vi "Format String to Numeric.vi"(4 "Response":string, 5 "Ignore String":string, 6 "Type":T2, 7 "Data Parameters.List":string[](array[string]), 8 "error in (no error)":errorcluster, 9 "Channel Type":T1, 10 "Format String":string, 11 "Expected String":string) -> (0 "error out":errorcluster, 2 "Value":dbl, 3 "remaining string":string)   [LabVIEW 2013, in "Instrument Addon Engine.lvlib"]
uses:
  Instrument Addon Engine.lvlib
  Shared/Types/Type Cast Type.ctl
  Shared/Types/Data Channel Type.ctl
  Shared/Instrument Addon Shared.lvlib
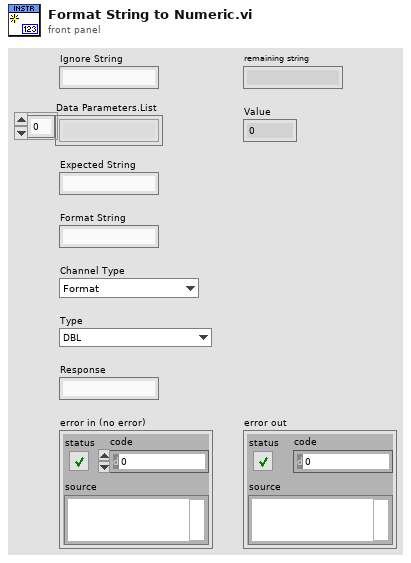
[diagram p1: front panel]
types:
  T1 = typedef "Instrument Addon Shared.lvlib/Data Channel Type.ctl" = enum16{"Format", "Comparison", "Type Cast", "Enumerated List"}
  T2 = typedef "Instrument Addon Shared.lvlib/Type Cast Type.ctl" = enum16{"DBL", "SGL", "U64", "U32", "U16", "U8", "I64", "I32", "I16", "I8"}
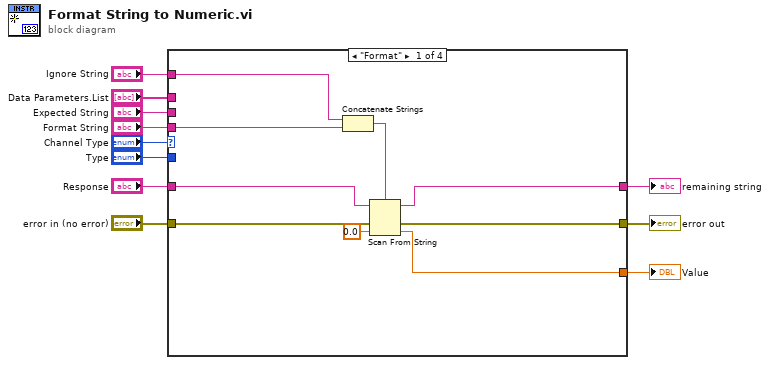
[diagram p0: block diagram]
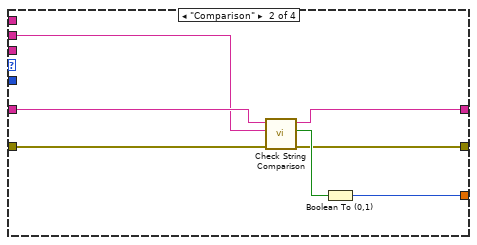
[diagram p2: hidden frame]
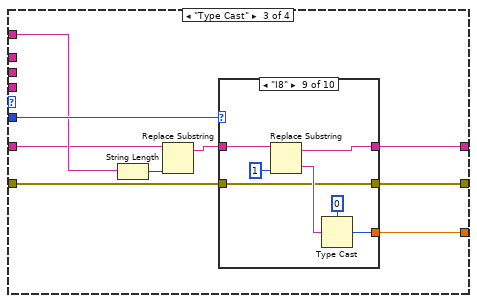
[diagram p3: hidden frame]
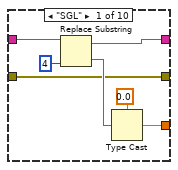
[diagram p4: hidden frame]
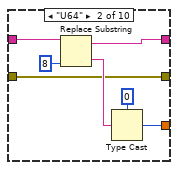
[diagram p5: hidden frame]
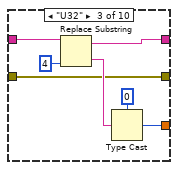
[diagram p6: hidden frame]
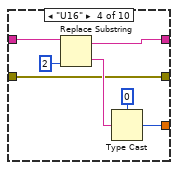
[diagram p7: hidden frame]
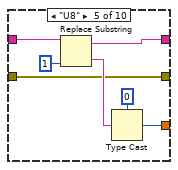
[diagram p8: hidden frame]
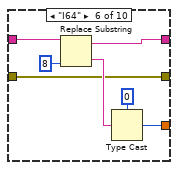
[diagram p9: hidden frame]
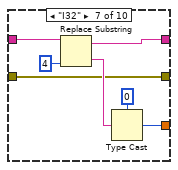
[diagram p10: hidden frame]
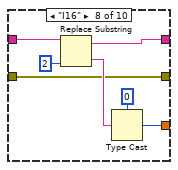
[diagram p11: hidden frame]
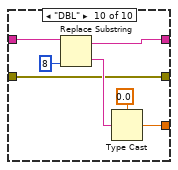
[diagram p12: hidden frame]
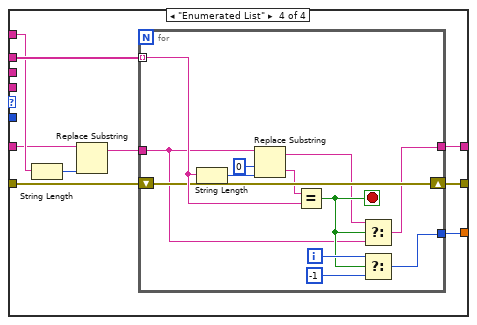
[diagram p13: hidden frame]
diagram:
  n1 = case shown="\"Format\"" "Channel Type" {
    tunnel: [w19 w27 w35 w113] -> w9
    tunnel: "Response" -> [w20 w26 w31 w108]
    tunnel: [w18 w24 w36 w111] -> w3
    tunnel: "Ignore String" -> [w16 _ w32 w109]
    tunnel: "Format String" -> [w15 _ _ _]
    tunnel: "error in (no error)" -> [w14 w22 w29 w115]
    tunnel: [w13 w21 w33 w112] -> w6
    tunnel: "Expected String" -> [_ w25 _ _]
    tunnel: "Type" -> [_ _ w34 _]
    tunnel: "Data Parameters.List" -> [_ _ _ w114]
    frame "Format" {
      n2 = Concatenate Strings(w16, w15) -> (w12:string)
      n3 = Scan From String(format string=w12, input string=w20, error in=w14, default 1=0.0 ("default value 1")) -> (remaining string=w18:string, error out=w13:errorcluster, output 1=w19:dbl)  [unwired: 1 in, 1 out]
    }
    frame "Comparison" {
      n4 = call "Check String Comparison.vi"("error in (no error)"=w22, "Expected String"=w25, "String"=w26) -> ("error out"=w21:errorcluster, "Found?"=w23:bool, "string out"=w24:string)  [unwired: 6 in]
      n5 = Boolean To (0,1)(Boolean=w23) -> (0, 1=w27:i16)
    }
    frame "Type Cast" {
      n6 = String Length(string=w32) -> (length=w28:i32)
      n7 = Replace Substring(2:w28, 5:w31) -> (1:w30:string)  [unwired: 2 in, 1 out]
      n8 = case shown="\"I8\"" w34 {
        tunnel: w30 -> [w43 w50 w57 w64 w71 w78 w85 w92 w99 w106]
        tunnel: [w42 w49 w56 w63 w70 w77 w84 w91 w98 w105] -> w36
        tunnel: [w38 w45 w52 w59 w66 w73 w80 w87 w94 w101] -> w35
        tunnel: [w37 w44 w51 w58 w65 w72 w79 w86 w93 w100] -> w33
        tunnel: w29 -> [w37 w44 w51 w58 w65 w72 w79 w86 w93 w100]
        frame "SGL" {
          n9 = Replace Substring(2:4 ("length (len. of substring)"), 5:w43) -> (0:w40:string, 1:w42:string)  [unwired: 2 in]
          n10 = Type Cast(type=sgl 0.0, x=w40) -> (*(type *) &x=w38:sgl)
        }
        frame "U64" {
          n11 = Replace Substring(2:8 ("length (len. of substring)"), 5:w50) -> (0:w47:string, 1:w49:string)  [unwired: 2 in]
          n12 = Type Cast(type=u64 0, x=w47) -> (*(type *) &x=w45:u64)
        }
        frame "U32" {
          n13 = Replace Substring(2:4 ("length (len. of substring)"), 5:w57) -> (0:w54:string, 1:w56:string)  [unwired: 2 in]
          n14 = Type Cast(type=u32 0, x=w54) -> (*(type *) &x=w52:u32)
        }
        frame "U16" {
          n15 = Replace Substring(2:2 ("length (len. of substring)"), 5:w64) -> (0:w61:string, 1:w63:string)  [unwired: 2 in]
          n16 = Type Cast(type=u16 0, x=w61) -> (*(type *) &x=w59:u16)
        }
        frame "U8" {
          n17 = Replace Substring(2:1 ("length (len. of substring)"), 5:w71) -> (0:w68:string, 1:w70:string)  [unwired: 2 in]
          n18 = Type Cast(type=u8 0, x=w68) -> (*(type *) &x=w66:u8)
        }
        frame "I64" {
          n19 = Replace Substring(2:8 ("length (len. of substring)"), 5:w78) -> (0:w75:string, 1:w77:string)  [unwired: 2 in]
          n20 = Type Cast(type=i64 0, x=w75) -> (*(type *) &x=w73:i64)
        }
        frame "I32" {
          n21 = Replace Substring(2:4 ("length (len. of substring)"), 5:w85) -> (0:w82:string, 1:w84:string)  [unwired: 2 in]
          n22 = Type Cast(type=0, x=w82) -> (*(type *) &x=w80:i32)
        }
        frame "I16" {
          n23 = Replace Substring(2:2 ("length (len. of substring)"), 5:w92) -> (0:w89:string, 1:w91:string)  [unwired: 2 in]
          n24 = Type Cast(type=i16 0, x=w89) -> (*(type *) &x=w87:i16)
        }
        frame "I8" {
          n25 = Replace Substring(2:1 ("length (len. of substring)"), 5:w99) -> (0:w96:string, 1:w98:string)  [unwired: 2 in]
          n26 = Type Cast(type=i8 0, x=w96) -> (*(type *) &x=w94:i8)
        }
        frame "DBL" {
          n27 = Replace Substring(2:8 ("length (len. of substring)"), 5:w106) -> (0:w103:string, 1:w105:string)  [unwired: 2 in]
          n28 = Type Cast(type=0.0, x=w103) -> (*(type *) &x=w101:dbl)
        }
      }
    }
    frame "Enumerated List" {
      n29 = String Length(string=w109) -> (length=w110:i32)
      n30 = Replace Substring(2:w110, 5:w108) -> (1:w107:string)  [unwired: 2 in, 1 out]
      n31 = for {
        shift-right: [w123] -> w112
        shift-left: w115 -> [w123]
        tunnel: w114 -> [w127] mode=indexing
        tunnel: w107 -> [w118]
        tunnel: [w124] -> w113
        tunnel: [w116] -> w111
        i -> [w126]
        stop <- w119 stop-if-true
        n32 = String Length(string=w127) -> (length=w122:i32)
        n33 = Replace Substring(2:w122, 3:0 ("offset (0)"), 5:w118) -> (0:w120:string, 1:w117:string)  [unwired: 1 in]
        n34 = Equal?(x=w120, y=w127) -> (x = y?=w119:bool)
        n35 = Select(t=w117, s=w119, f=w118) -> (s? t:f=w116:string)
        n36 = Select(t=w126, s=w119, f=-1) -> (s? t:f=w124:i32)
      }
    }
  }
  "Value" <- w9
  "error out" <- w6
  "remaining string" <- w3
